vi "DeppPutRegSet.vi"(7 "Overlap?":bool, 8 "Error In":errorcluster, 9 "Data":u8[](array[numeric]), 10 "Addresses":u8[](array[numeric]), 11 "Device Handle":u32) -> (0 "Error Out":errorcluster, 3 "Device Handle":u32)   [LabVIEW 2011, in "LVH-Adept.lvlib" / "DEPP.lvlib"]
uses:
  DEPP.lvlib
  Private/Type Defs/Error.ctl
  depp.dll
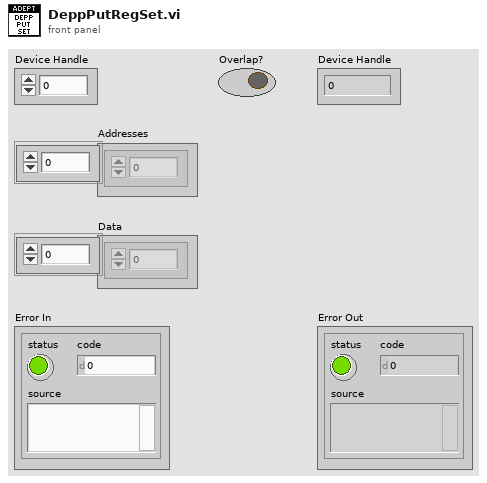
[diagram p1: front panel]
types:
  T1 = typedef "LVH-Adept.lvlib/DEPP.lvlib/Error.ctl" = enum16{"Unknown", "Enable", "Enable Port", "Get Register", "Get Register Repeat", "Get Register Set", "Put Register", "Put Register Repeat", "Put Register Set", "Disable", "Set Pair Size"}
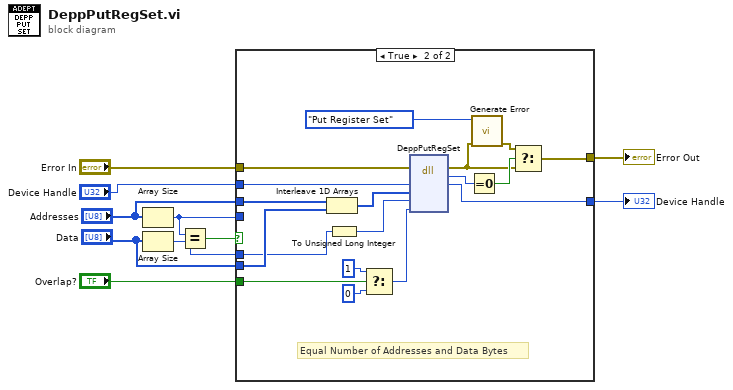
[diagram p0: block diagram]
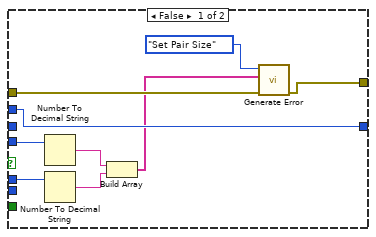
[diagram p2: hidden frame]
diagram:
  n1 = Array Size(array="Addresses") -> (size(s)=w2:i32)
  n2 = Array Size(array="Data") -> (size(s)=w1:i32)
  n3 = Equal?(x=w2, y=w1) -> (x = y?=w5:bool)
  n4 = case shown="True" w5 {
    tunnel: "Error In" -> [w18 w37]
    tunnel: [w17 w34] -> w9
    tunnel: [w19 w33] -> w8
    tunnel: "Device Handle" -> [w19 w32]
    tunnel: "Overlap?" -> [_ w28]
    tunnel: "Addresses" -> [_ w23]
    tunnel: "Data" -> [_ w22]
    tunnel: w2 -> [w15 _]
    tunnel: w1 -> [w16 w21]
    frame False {
      n5 = Number To Decimal String(number=w15) -> (decimal integer string=w14:string)  [unwired: 1 in]
      n6 = Number To Decimal String(number=w16) -> (decimal integer string=w13:string)  [unwired: 1 in]
      n7 = Build Array(w14, w13) -> (w12:string[])
      n8 = call "Generate Error.vi"("Error In"=w18, "Arguments"=w12, "DEPP Error"=Error."Set Pair Size") -> ("Error Out"=w17:errorcluster)  [unwired: 8 in]
    }
    frame True {
      # "Equal Number of Addresses and Data Bytes"
      n9 = Interleave 1D Arrays(w23, w22) -> (w24:u8[])
      n10 = To Unsigned Long Integer(number=w21) -> (unsigned 32bit integer=w20:u32)
      n11 = Select(t=u8 1, s=w28, f=u8 0) -> (s? t:f=w25:u8)
      n12 = dll-call lib="depp.dll" fn="DeppPutRegSet"(error in=w37, "hif"=w32, "pbAddrData"=w24, "nAddrDataPairs"=w20, "fOverlap"=w25) -> (error out=w29:errorcluster, "Success"=w36:u32, "hif"=w33:u32)  [unwired: 5 in, 1 out]
      n13 = Equal To 0?(x=w36) -> (x = 0?=w35:bool)
      n14 = call "Generate Error.vi"("Error In"=w29, "DEPP Error"=Error."Put Register Set") -> ("Error Out"=w30:errorcluster)  [unwired: 9 in]
      n15 = Select(t=w30, s=w35, f=w29) -> (s? t:f=w34:errorcluster)
    }
  }
  "Error Out" <- w9
  "Device Handle" <- w8
